vi "Listener Async.vi"(9 "Endpoint":refnum<class "Endpoint.lvclass">, 10 "Listener Notifier":T1, 11 "Listener":refnum<k5>) -> ()   [LabVIEW 2020, in "Stream-TCP.lvlib" / "TCP Client.lvclass"]
uses:
  TCP Client.lvclass
  Listener Notifier.ctl
  Listener Result.ctl
  Listener Status.ctl
  C:/Program Files (x86)/National Instruments/LabVIEW 2020/vi.lib/IlluminatedG/lv-stream/Connection/Connection.lvclass
  <vilib>/IlluminatedG/lv-stream/Endpoint/Endpoint.lvclass
  <vilib>/IlluminatedG/lv-stream/Connection State.ctl
  Stream-TCP.lvlib
  <vilib>/IlluminatedG/lv-stream/Connection/Connection.lvclass
  <vilib>/IlluminatedG/lv-stream/Stream.lvlib
  <vilib>/IlluminatedG/lv-stream/URI/URI.lvclass
panel:
  out "Local URI":string
  out "URI String":string
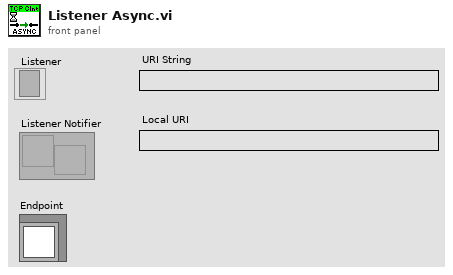
[diagram p1: front panel]
types:
  T1 = typedef "Stream-TCP.lvlib/Listener Notifier.ctl" = refnum<notifier>
  T2 = typedef "Stream-TCP.lvlib/Listener Result.ctl" = cluster{"Status":T3, "Client":refnum<class "TCP Client.lvclass">, "Ack Notifier":refnum<notifier>}
  T3 = typedef "Stream-TCP.lvlib/Listener Status.ctl" = enum16{"Successful", "Unsuccessful"}
  T4 = typedef "Stream.lvlib/Connection State.ctl" = enum16{"Connected", "Disconnected"}
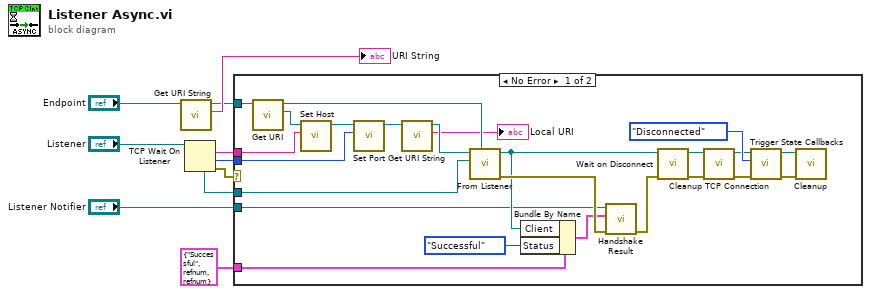
[diagram p0: block diagram]
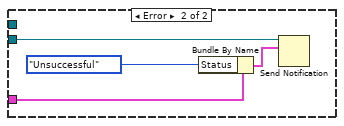
[diagram p2: hidden frame]
diagram:
  n1 = call <vilib>:"Get URI String.vi"("Endpoint in"="Endpoint") -> ("URI String"=→"URI String":string, "Endpoint out"=w2:refnum<class "Endpoint.lvclass">)  [unwired: 8 in, 1 out]
  n2 = TCP Wait On Listener(11:"Listener") -> (0:w7:errorcluster, 1:w4:u16, 2:w5:string, 4:w6:refnum<k5>)  [unwired: 3 in, 1 out]
  n3 = case shown="No Error" w7 {
    tunnel: w6 -> [w33 _]
    tunnel: w5 -> [w27 _]
    tunnel: w4 -> [w25 _]
    tunnel: "Listener Notifier" -> [w16 w38]
    tunnel: w2 -> [w29 _]
    tunnel: T2 {"Status"=enum."Successful", "Client"=refnum, "Ack Notifier"=refnum} ("Result") -> [w21 w37]
    frame No Error {
      n4 = call <vilib>:"Get URI.vi"("Endpoint in"=w29) -> ("URI"=w28:refnum<class "URI.lvclass">, "Endpoint out"=w24:refnum<class "Endpoint.lvclass">)  [unwired: 8 in, 1 out]
      n5 = call <vilib>:"Set Host.vi"("Host"=w27, "URI in"=w28) -> ("URI out"=w26:refnum<class "URI.lvclass">)  [unwired: 8 in, 1 out]
      n6 = call <vilib>:"Set Port.vi"("Port"=w25, "URI in"=w26) -> ("URI out"=w13:refnum<class "URI.lvclass">)  [unwired: 8 in, 1 out]
      n7 = call <vilib>:"Get URI String.vi"("URI in"=w13) -> ("URI String"=→"Local URI":string, "URI out"=w12:refnum<class "URI.lvclass">)  [unwired: 8 in, 1 out]
      n8 = call "From Listener.vi"("From"=w24, "TCP Connection"=w33, "URI"=w12) -> ("error out"=w34:errorcluster, "TCP Client"=w23:refnum<class "TCP Client.lvclass">)  [unwired: 7 in]
      n9 = Bundle By Name(cluster=w21, "Client"=w23, "Status"=Listener_Status."Successful") -> (w15:T2)
      n10 = call "Handshake Result.vi"("error in (no error)"=w34, "Result"=w15, "Listener Notifier"=w16) -> ("error out"=w14:errorcluster)  [unwired: 8 in]
      n11 = call "Wait on Disconnect.vi"("error in (no error)"=w14, "TCP Client in"=w23) -> ("error out"=w19:errorcluster, "TCP Client out"=w20:refnum<class "TCP Client.lvclass">)  [unwired: 8 in]
      n12 = call "Cleanup TCP Connection.vi"("error in (no error)"=w19, "TCP Client in"=w20) -> ("error out"=w18:errorcluster, "TCP Client out"=w17:refnum<class "TCP Client.lvclass">)  [unwired: 8 in]
      n13 = call <vilib>:"Trigger State Callbacks.vi"("error in (no error)"=w18, "State"=Connection_State."Disconnected", "Connection in"=w17) -> ("error out"=w31:errorcluster, "Connection out"=w30:refnum<class "TCP Client.lvclass">)  [unwired: 7 in]
      n14 = call-dynamic "Cleanup.vi"("error in (no error)"=w31, "TCP Client in"=w30) -> ()  [unwired: 9 in, 1 out]
    }
    frame Error {
      n15 = Bundle By Name(cluster=w37, "Status"=Listener_Status."Unsuccessful" ("notification")) -> (w35:T2)
      n16 = Send Notification(notification=w35, notifier=w38) -> ()  [unwired: 1 in, 2 out]
    }
  }
